vi "BG1FGV.vi"(8 "Error In":errorcluster, 10 "action":enum16{"write", "read"}(ring)=enum."read", 11 "BG1 in":dbl[](array[numeric])) -> (0 "Error Out":errorcluster, 3 "BG1 out":dbl[](array[numeric]))   [LabVIEW 2020]
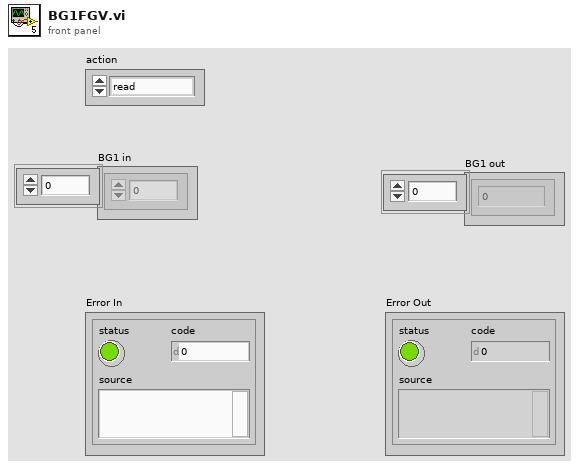
[diagram p1: front panel]
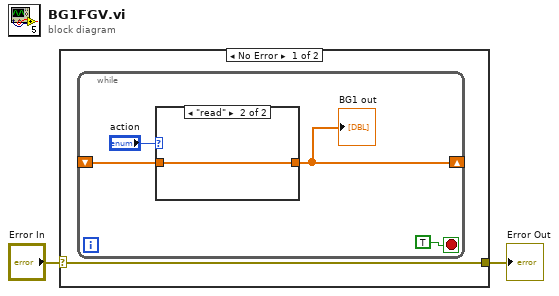
[diagram p0: block diagram]
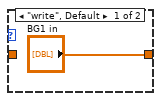
[diagram p2: hidden frame]
diagram:
  n1 = case shown="No Error" "Error In" {
    selector: "Error In" -> [w3 w10]
    tunnel: [w3 w10] -> w1
    frame No Error {
      n2 = while {
        shift-right: [w6] -> _
        shift-left: _ -> [w4]
        stop <- TRUE stop-if-true
        n3 = case shown="\"read\"" "action" {
          tunnel: ["BG1 in" w9] -> w6
          tunnel: w4 -> [_ w9]
          frame "write", Default {
          }
          frame "read" {
          }
        }
        "BG1 out" <- w6
      }
    }
    frame Error {
    }
  }
  "Error Out" <- w1
